vi "getFrame.vi"(0 "numOfFrame":u16) -> (1 "return type":i32, 2 "framePixelsBuffer":u16[](array[numeric]))   [LabVIEW 2012]
uses:
  hidapi_32bits.dll
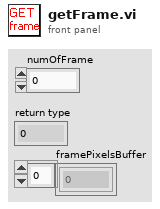
[diagram p1: front panel]
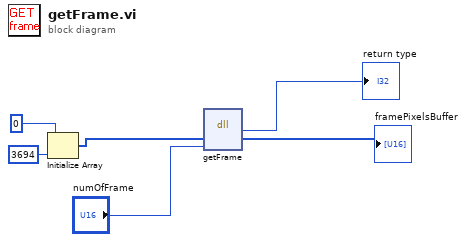
[diagram p0: block diagram]
diagram:
  n1 = Initialize Array(u16 0 ("element"), 3694 ("dimension size")) -> (w4:u16[])
  n2 = dll-call lib="C:/All_Data/mikrocont/Project1/New_controller__Jan_2015/LabView_Aug_2015/hidapi_32bits.dll" fn="getFrame"("framePixelsBuffer"=w4, "numOfFrame"="numOfFrame") -> ("return type"=→"return type":i32, "framePixelsBuffer"=→"framePixelsBuffer":u16[])  [unwired: 4 in, 2 out]
